vi "SIAM_spielerein.vi"() -> ()   [LabVIEW 2011]
uses:
  SIAM_command.ctl
panel:
  in  "command 2":T1=4027514895 format="%x" items=["read_x-Motor_status_ticket"=17305600, "init_x-Motor"=17760263, "read_x-Motor_absolute_ticket"=16781312, "move_x-Motor_absolute"=16777217, "move_x-Motor_relative"=16842753, "read_y-Motor_status_ticket"=18354176, "init_y-Motor"=18808839, "read_y-Motor_absolute_ticket"=17829888, "move_y-Motor_absolute"=17825793, "move_y-Motor_relative"=17891329, "read_z-Motor_status_ticket"=19402752, "init_z-Motor"=19857415, "stop_z-Motor"=19857423, "start_z-Motor"=19857422, "read_z-Motor_absolute_ticket"=18878464, "move_z-Motor_absolute"=18874369, "move_z-Motor_relative"=18939905, "end_no_ticket"=4027514895, "end_ticket"=4027518991, "IO-read_bank0"=218107904, "IO-write_bank0"=218103809, "IO-read_bank1"=219156480, "IO-write_bank1"=219152385, "IO-delay_bank0"=218365953, "IO-delay_bank0_fromVar"=218365955, "read_cam_clock"=3289124864, "store_cam_clock"=3289120770, "read_cam_phase"=3289190400, "set_cam_deadtime"=3288989697, "set_cam_10uscycles"=3289055233, "set_cam_10uscycles_fromVariable"=3289055235, "calc_cam"=3289317386, "store_cam_Var"=3289251842, "math_addToVariable"=4060086278, "readVar"=4060090368, "writeVar"=4060086273, "copyVar"=4060086276, "decrement_branchRel_if_equal"=4043374945, "decrement_branchRel_if_greaterequal"=4043375201, "decrement_branchRel_if_greaterequal_withTicket"=4043379297, "decrement_branchRel_if_smaller"=4043375457, "increment_branchRel_if_smaller"=4043375473, "set_x-Galvo"=102760689, "set_y-Galvo"=103809265, "set_z-Fokus"=104857841, "read_x-Galvo_ticket"=102764608, "read_y-Galvo_ticket"=103813184, "read_z-Focus_ticket"=104861760, "x-Galvo_pos_fromVar"=102760515, "y-Galvo_pos_fromVar"=103809091, "z-Focus_pos_fromVar"=104857667]
  in  "Type":enum8{"acc", "vel", "abs", "offset"}(ring)
  in  "ResolutionBits":dbl[][](array[numeric])
  out "x = y? 2":bool
  out "error out":errorcluster
  out "x = y?":bool
  in  "connection ID":refnum<k5>
  out "log2(x)":dbl
  in  "Numeric 2":u32 format="%.0x"
  out "x*2^n":dbl
  out "y":i32
  in  "Numeric":dbl
  in  "ResolutionBits":u8
  in  "command":u32(ring)=4027514895 format="%x" items=["read_x-Motor_status_ticket"=17305600, "init_x-Motor"=17760263, "read_x-Motor_absolute_ticket"=16781312, "move_x-Motor_absolute"=16777217, "move_x-Motor_relative"=16842753, "read y-Motor status, ticket"=18354176, "init y-Motor"=18808839, "read y-Motor absolute, ticket"=17829888, "move y-Motor absolute"=17825793, "move y-Motor relative"=17891329, "read z-Motor status, ticket"=19402752, "init z-Motor"=19857415, "stop z-Motor"=19857423, "start z-Motor"=19857422, "read z-Motor absolute, ticket"=18878464, "move z-Motor absolute"=18874369, "move z-Motor relative"=18939905, "end_no_ticket"=4027514895, "end_ticket"=4027518991, "IO-read_bank0"=218107904, "IO-write_bank0"=218103809, "IO-read_bank1"=219156480, "IO-write_bank1"=219152385, "IO-delay_bank0"=218365953, "IO-delay_bank0_fromVar"=218365955, "read_cam_clock"=3289124864, "set_cam_deadtime"=3288989697, "set_cam_10uscycles"=3289055233, "calc_cam"=3289317386, "store_cam_Var"=3289251842, "math_substractFromVariable"=4060086278, "readVar"=4060090368, "writeVar"=4060086273, "copyVar"=4060086276, "decrement_branchRel_if_greater"=4043374945, "decrement_branchRel_if_greaterequal"=4043375201, "writeTMSI"=100663297, "writeTMSI_fromVar"=100663299]
  out "Descriptions":cluster{u32, "ValueText":string}[](array[cluster])=[{17305600, "ValueText"="read status of x-motor, 0=ON_AND_NOT_INIT, 1=ON_AND_INIT, 3=offandinit"}, {17760263, "ValueText"="init x-motor, needs some seconds"}, {16781312, "ValueText"="read x-Motor absolute position in uSteps"}, {16777217, "ValueText"="x-Motor write absolute position in uSteps"}, {16842753, "ValueText"="x-Motor write relative position in uSteps"}, {18354176, "ValueText"="read status of y-motor, 0=ON_AND_NOT_INIT, 1=ON_AND_INIT, 3=offandinit"}, {18808839, "ValueText"="init y-motor, needs some seconds"}, {17829888, "ValueText"="read y-Motor absolute position in uSteps"}, {17825793, "ValueText"="y-Motor write absolute position in uSteps"}, {17891329, "ValueText"="y-Motor write relative position in uSteps"}, {19402752, "ValueText"="read status of z-motor, 0=ON_AND_NOT_INIT, 1=ON_AND_INIT, 3=offandinit"}, {19857415, "ValueText"="init z-motor, needs some seconds"}, {19857423, "ValueText"="stop z-motor, go out of closed loop"}, {19857422, "ValueText"="start z-motor, go into closed loop"}, {18878464, "ValueText"="read z-Motor absolute position in uSteps"}, {18874369, "ValueText"="z-Motor write absolute position in uSteps"}, {18939905, "ValueText"="z-Motor write relative position in uSteps"}, {4027514895, "ValueText"="end without ticket"}, {4027518991, "ValueText"="end with ticket"}, {218107904, "ValueText"="IO-read_bank0"}, {218103809, "ValueText"="IO-write_bank0"}, {218365953, "ValueText"="next bank0 with highres delay"}, {218365955, "ValueText"="next bank0 with highres delay, value from variable"}, {3289124864, "ValueText"="read background-measured 100MHz ticks between 256 camclocks"}, {3288989697, "ValueText"="set delay in 100MHz ticks to avoid small result, avoid trigger problems, 100"}, {3289055233, "ValueText"="set future 10µs cycels to calculate modulo"}, {3289251842, "ValueText"="store modulo result in user variable n"}, {4060090368, "ValueText"="read variable n"}, {4060086273, "ValueText"="set variable n"}, {4060086276, "ValueText"="copy variable m to n"}, {4043374945, "ValueText"="decrement and branch if greater"}, {4043375201, "ValueText"="decrement and branch if greater or equal"}, {100663297, "ValueText"="write TMSI,TMSI-order,data"}, {100663299, "ValueText"="write TMSI,from variable"}] {"?" format="%.0x"}
  out "value":i32=120 format="%.0b"
  in  "I16:16":fxp<+/-,32,16> format="%.2p"
  in  "#Entries":i32
  in  "Script":T2(array[cluster])=[{"command"=4027514895, "Delay 10µs"=0, "P0"=16777215, "P1"=0, "P2"=0, "P3"=0, "P4"=0, "P5-ticket"=0}, {"command"=4027514895, "Delay 10µs"=0, "P0"=100, "P1"=0, "P2"=0, "P3"=0, "P4"=0, "P5-ticket"=0}, {"command"=4027514895, "Delay 10µs"=0, "P0"=5, "P1"=120, "P2"=0, "P3"=0, "P4"=0, "P5-ticket"=0}] {"command" format="%x" items=["read_x-Motor_status_ticket"=17305600, "init_x-Motor"=17760263, "read_x-Motor_absolute_ticket"=16781312, "move_x-Motor_absolute"=16777217, "move_x-Motor_relative"=16842753, "read y-Motor status, ticket"=18354176, "init y-Motor"=18808839, "read y-Motor absolute, ticket"=17829888, "move y-Motor absolute"=17825793, "move y-Motor relative"=17891329, "read z-Motor status, ticket"=19402752, "init z-Motor"=19857415, "stop z-Motor"=19857423, "start z-Motor"=19857422, "read z-Motor absolute, ticket"=18878464, "move z-Motor absolute"=18874369, "move z-Motor relative"=18939905, "end_no_ticket"=4027514895, "end_ticket"=4027518991, "IO-read_bank0"=218107904, "IO-write_bank0"=218103809, "IO-read_bank1"=219156480, "IO-write_bank1"=219152385, "IO-delay_bank0"=218365953, "IO-delay_bank0_fromVar"=218365955, "read_cam_clock"=3289124864, "set_cam_deadtime"=3288989697, "set_cam_10uscycles"=3289055233, "calc_cam"=3289317386, "store_cam_Var"=3289251842, "math_substractFromVariable"=4060086278, "readVar"=4060090368, "writeVar"=4060086273, "copyVar"=4060086276, "decrement_branchRel_if_greater"=4043374945, "decrement_branchRel_if_greaterequal"=4043375201, "writeTMSI"=100663297, "writeTMSI_fromVar"=100663299]}
  in  "allow movement from end":i32
  in  "allowed start movement":i32
  in  "max. Estimate/Deterministic":bool
  in  "Duration Ticks":i32
  in  "Fixed Base Adress (<>0)":dbl
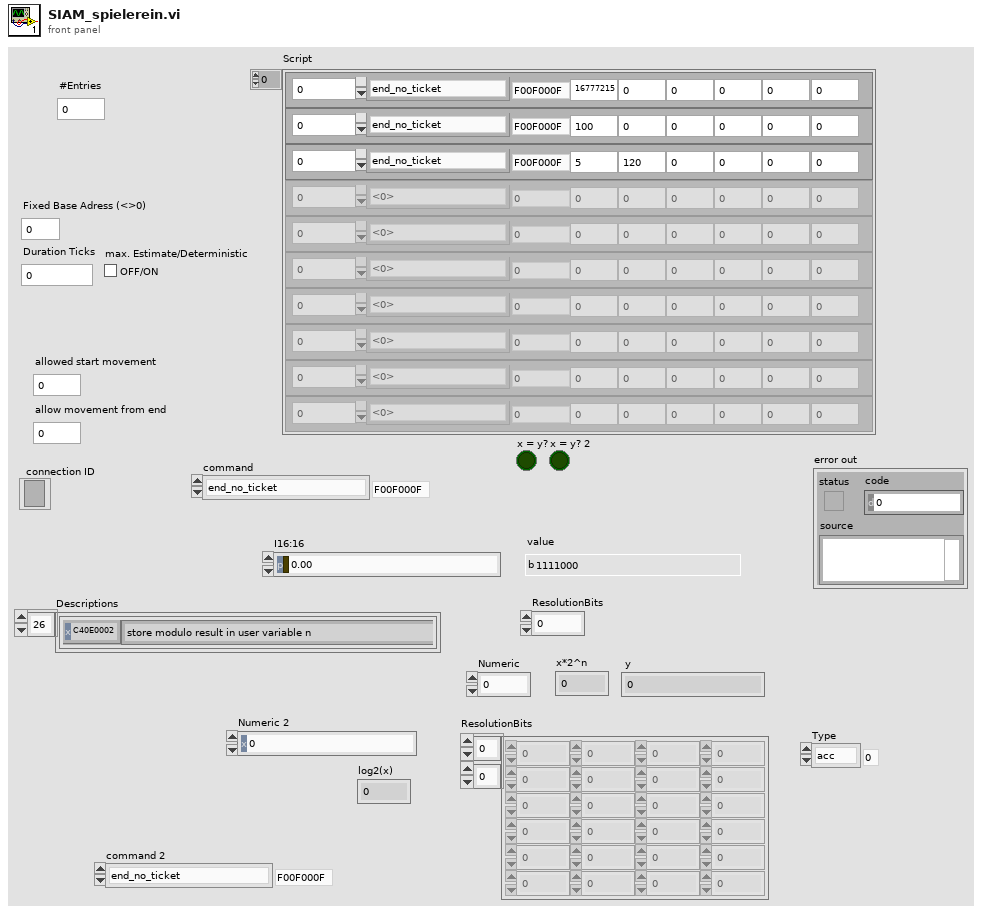
[diagram p1: front panel]
types:
  T1 = typedef "SIAM_command.ctl" = u32
  T2 = cluster{"command":u32, "Delay 10µs":u32, "P0":i32, "P1":i32, "P2":i32, "P3":i32, "P4":i32, "P5-ticket":i32}[]
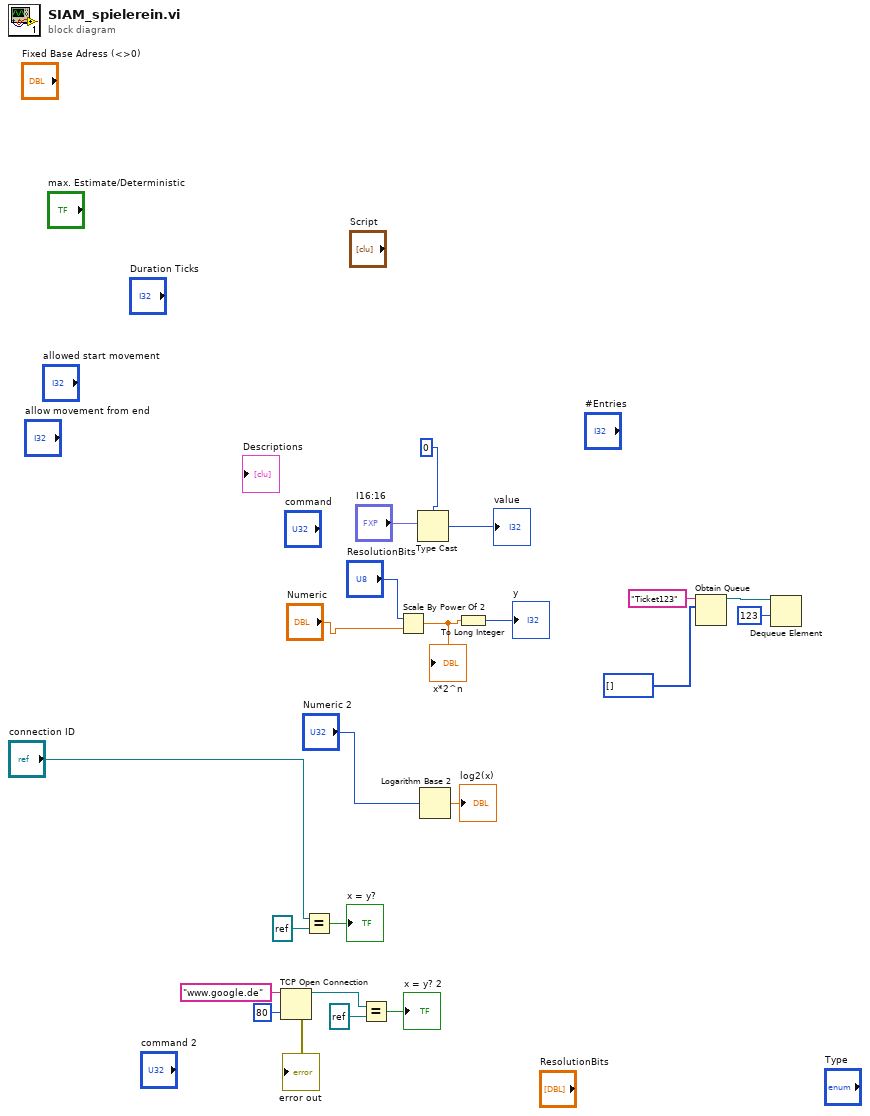
[diagram p0: block diagram]
diagram:
  n1 = TCP Open Connection(address="www.google.de", remote port or service name=u16 80) -> (connection ID=w5:refnum<k5>, error out=→"error out":errorcluster)  [unwired: 3 in]
  n2 = Equal?(x="connection ID", y=refnum<k5> refnum) -> (x = y?=→"x = y?":bool)
  n3 = Equal?(x=w5, y=refnum<k5> refnum) -> (x = y?=→"x = y? 2":bool)
  n4 = Scale By Power Of 2(n="ResolutionBits", x="Numeric") -> (x*2^n=w17:dbl)
  "x*2^n" <- w17
  n5 = Type Cast(type=i64 0, x="I16:16") -> (*(type *) &x=→"value":i64)
  n6 = Logarithm Base 2(1:"Numeric 2") -> (0:→"log2(x)":dbl)
  n7 = To Long Integer(number=w17) -> (32bit integer=→"y":i32)
  n8 = Obtain Queue(name (unnamed)="Ticket123", element data type=i32[] []) -> (queue out=w13:refnum<queue>)  [unwired: 3 in, 2 out]
  n9 = Dequeue Element(queue=w13, timeout in ms (-1)=123) -> ()  [unwired: 1 in, 4 out]
